vi "Get Timer.vi"(2 "Mode":enum8{"Start", "Get"}(ring), 5 "Timeout(ms)":u32=1000) -> (0 "Timeout ?":bool, 1 "Time(ms)":u32)   [LabVIEW 2015, in "KEYENCE LJ-X8000A.lvlib"]
uses:
  KEYENCE LJ-X8000A.lvlib
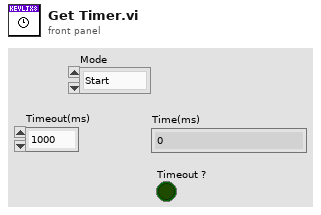
[diagram p1: front panel]
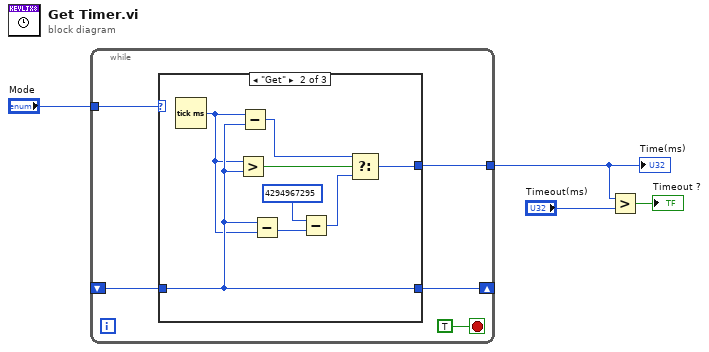
[diagram p0: block diagram]
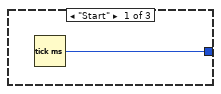
[diagram p2: hidden frame]
diagram:
  n1 = while {
    tunnel: "Mode" -> [w9]
    shift-right: [w8] -> _
    shift-left: _ -> [w7]
    tunnel: [w6] -> w3
    stop <- TRUE stop-if-true
    n2 = case shown="\"Get\"" w9 {
      tunnel: [w10 w16 w19] -> w8
      tunnel: w7 -> [_ w16 w19]
      tunnel: [_ w11 _] -> w6
      frame "Start" {
        n3 = Tick Count (ms)() -> (millisecond timer value=w10:u32)
      }
      frame "Get" {
        n4 = Tick Count (ms)() -> (millisecond timer value=w15:u32)
        n5 = Greater?(x=w15, y=w16) -> (0:w18:bool)
        n6 = Subtract(x=w15, y=w16) -> (x-y=w17:u32)
        n7 = Subtract(x=w16, y=w15) -> (x-y=w13:u32)
        n8 = Subtract(x=u32 4294967295, y=w13) -> (x-y=w12:u32)
        n9 = Select(t=w17, s=w18, f=w12) -> (s? t:f=w11:u32)
      }
      frame Default {
      }
    }
  }
  "Time(ms)" <- w3
  n10 = Greater?(x=w3, y="Timeout(ms)") -> (0:→"Timeout ?":bool)
